vi "Fire HIL Shot.vi"(8 "error in":errorcluster) -> (0 "error out":errorcluster, 1 "Shot Completed":bool)   [LabVIEW 2017, in "DTACQ - Network Enabled Device Driver.lvlib"]
doc: "Connects to the appropriate port, in order to cause a shot to be fired."
uses:
  DTACQ - Network Enabled Device Driver.lvlib
  Communications/Typedefs/Functional Global Variable Action--Enum.ctl
  Communications/Communications Library.lvlib
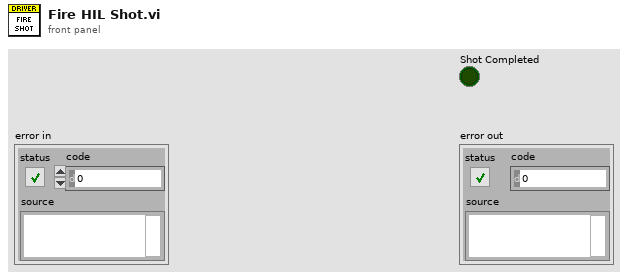
[diagram p1: front panel]
types:
  T1 = typedef "Communications Library.lvlib/Functional Global Variable Action--Enum.ctl" = enum16{"Initialise", "Write Module Config", "Write Carrier Config", "Read"}
  T2 = typedef "Communications Library.lvlib/DTACQ Module Carrier Configuration--Cluster.ctl" = cluster{"Name":string, "IP":string, "Control Port":i32, "Timeout (ms)":i32, "Continuous Capture Port (Multiplexed)":i32, "Start HIL Shot Port":i32, "AWG Upload Port (Multiplexed)":i32, "Download Captured Data Port (Multiplexed)":i32, "Module Slots":i32, "Module Configurations":T3[]}
  T3 = typedef "Communications Library.lvlib/DTACQ Module Configuration--Cluster.ctl" = cluster{"Name":string, "Position":string, "Module Type":T4, "Control Port":i32, "Timeout (ms)":i32, "Channels":i32}
  T4 = typedef "Communications Library.lvlib/DTACQ Device Type--Enum.ctl" = enum16{"Carrier", "Analog In Module", "Analog Out Module", "Generic Module"}
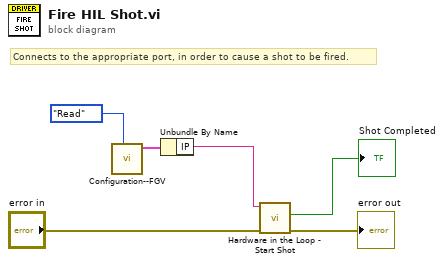
[diagram p0: block diagram]
diagram:
  # "Connects to the appropriate port, in order to cause a shot to be fired."
  n1 = call "Configuration--FGV.vi"("Functional Global Action"=Functional_Global_Variable_Action--Enum."Read") -> ("Carrier Configuration Out"=w5:T2)  [unwired: 9 in, 1 out]
  n2 = Unbundle By Name(w5) -> ("IP"=w4:string)
  n3 = call "Hardware in the Loop - Start Shot.vi"("error in"="error in", "Address"=w4) -> ("error out"=→"error out":errorcluster, "Shot Completed"=→"Shot Completed":bool)  [unwired: 8 in]
